vi "RemoveContained.vi"(8 "error in (no error)":errorcluster, 9 "Contained item path":string, 11 "CLabVIEWContainer in":refnum<class "CLabVIEWContainer.lvclass">) -> (0 "error out":errorcluster, 3 "CLabVIEWContainer out":refnum<class "CLabVIEWContainer.lvclass">)   [LabVIEW 2020, in "LabVIEWContainers.lvlib" / "CLabVIEWContainer.lvclass"]
uses:
  CLabVIEWContainer.lvclass
  CLabVIEWContainer.lvclass/CLabVIEWContainer.ctl
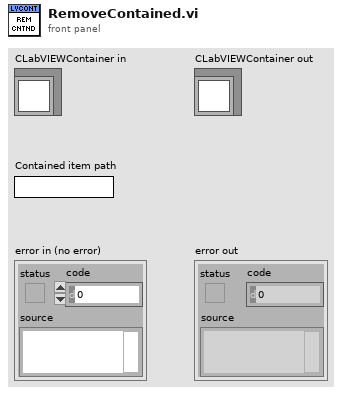
[diagram p1: front panel]
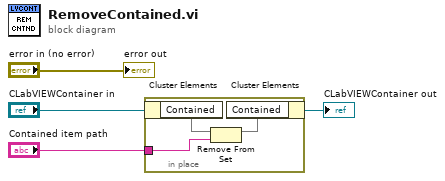
[diagram p0: block diagram]
diagram:
  n1 = in-place {
    in-place-border: "Contained item path" -> [w5]
    n2 = in-place-cluster #1("CLabVIEWContainer in") -> ("Contained"=w7:set{string})
    n3 = Remove From Set(10:w5, 11:w7) -> (3:w6:set{string})  [unwired: 1 out]
    n4 = in-place-cluster #1("Contained"=w6) -> (→"CLabVIEWContainer out":refnum<class "CLabVIEWContainer.lvclass">)
  }
  "error out" <- "error in (no error)"
